vi "DSF.Engine.Framework.Rx.Begin.vi"(8 "error in (no error)":errorcluster, 11 "Framework in":refnum<class "DSF.Engine.Framework.lvclass">) -> (0 "error out":errorcluster, 3 "Framework out":refnum<class "DSF.Engine.Framework.lvclass">)   [LabVIEW 2017, in "Data Sharing Framework Engine.lvlib" / "DSF.Engine.Framework.lvclass"]
uses:
  DSF.Engine.Framework.lvclass
  DSF.Engine.Framework.lvclass/DSF.Engine.Framework.ctl
  Status/DSF.Engine.Status.Framework.lvclass/DSF.Engine.Status.Framework.ctl
  Status/DSF.Engine.Status.Framework.Performance.lvclass/DSF.Engine.Status.Framework.Performance.ctl
  Status/DSF.Engine.Status.Framework.lvclass
  Status/DSF.Engine.Status.Framework.Performance.lvclass
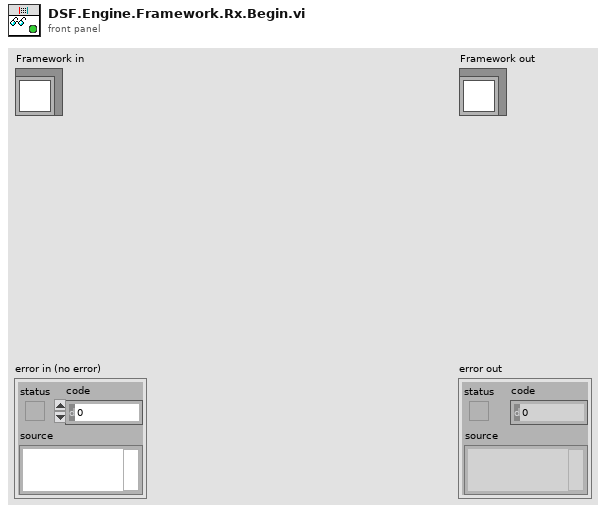
[diagram p1: front panel]
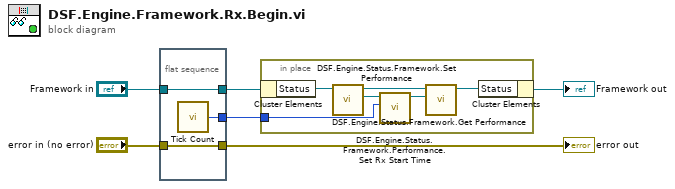
[diagram p0: block diagram]
diagram:
  n1 = flat-sequence {
    tunnel: "Framework in" -> [w8]
    tunnel: "error in (no error)" -> [w9]
    tunnel: [w9] -> w4
    tunnel: [w8] -> w3
    tunnel: [w7] -> w2
    frame #0 {
      n2 = call "Tick Count"() -> ("Tick Count(uSec)"=w7:u32)
    }
  }
  n3 = in-place {
    in-place-border: w2 -> [w10]
    n4 = in-place-cluster #1(w3) -> ("Status"=w15:refnum<class "DSF.Engine.Status.Framework.lvclass">)
    n5 = call "DSF.Engine.Status.Framework.Get Performance.vi"("Framework Status in"=w15) -> ("Framework Performance"=w14:refnum<class "DSF.Engine.Status.Framework.Performance.lvclass">, "Framework Status out"=w13:refnum<class "DSF.Engine.Status.Framework.lvclass">)  [unwired: 9 in]
    n6 = call "DSF.Engine.Status.Framework.Performance.Set Rx Start Time.vi"("Rx start time"=w10, "Framework Performance in"=w14) -> ("Framework Performance out"=w12:refnum<class "DSF.Engine.Status.Framework.Performance.lvclass">)  [unwired: 9 in]
    n7 = call "DSF.Engine.Status.Framework.Set Performance.vi"("Framework Performance"=w12, "Framework Status in"=w13) -> ("Framework Status out"=w11:refnum<class "DSF.Engine.Status.Framework.lvclass">)  [unwired: 9 in]
    n8 = in-place-cluster #1("Status"=w11) -> (→"Framework out":refnum<class "DSF.Engine.Framework.lvclass">)
  }
  "error out" <- w4
